vi "GUI_Scopes_NEW.vi"() -> ()   [LabVIEW 2020]
uses:
  Device Drivers/PXIdigitizer/subVis/Trigger.DigitalSource_TypDEf.ctl
  Device Drivers/ScopeAnalysis/SubVis/method_TypDef.ctl
  Device Drivers/ScopeAnalysis/SubVis/channels_TypDef.ctl
  Shared/GUI_Template/GUI_master/tcp new data cluster.ctl
  General-Controler/firstCall_TypDef.ctl
panel:
  in  "Trigger.Source::1":u16(ring) caption="Source"
  in  "Trigger.Coupling::1":u16(ring) caption="Coupling"
  in  "Analysis":T3={"Channel::1"=enum."Analysis1", "Calculations.Method::1"=enum."trigger", "Measurements::1"=-5e-07, "Calculations.Linked::1"=enum."na", "Calculations.Additional::1"=0.0} {"Calculations.Additional::1" min=0.0 max=0.0; "Measurements::1" min=0.0 max=0.0}
  in  "Horizontal.resolution::1":u16(ring) caption="Hres"
  in  "Horizontal.time_window::1":dbl=0.001 caption="TimeWindow" min=1e-09 max=100.0 format="%#_6p"
  in  "Horizontal.Min Sample Rate::1":dbl=500000000.0 caption="Sample Rate" min=1000.0 max=1000000000.0 step=1000000.0 format="%.0p"
  in  "Horizontal.Min Record Length::1":i32=1000 caption="Record Length" min=100 max=8388208 format="%.0p"
  in  "Trigger.Delay::1":dbl=0.5 caption="Delay" min=-10.0 max=10.0 format="%#_6p"
  in  "Trigger.Mode::1":u16(ring) caption="Mode"
  in  "Trigger.Low Level::1":dbl=0.5 caption="Level" min=-100.0 max=100.0 format="%#_6p"
  in  "Trigger.Slope::1":u16(ring) caption="Slope"
  in  "autoscale::1":bool caption="auto\nscale"
  in  "LocalSavingPath::1":path
  in  "save::1":bool=TRUE caption="save"
  in  "Select device":string(combo)="StagingPXIFast1"
  in  "Refresh Button":bool
  out "device status::1":string="Initialized" caption="Device status"
  in  "stop":bool=TRUE
  out "GUIdevice 1":string="StagingPXIFast1"
  in  "Waveform cluster":T4={"Channel::1"=enum."Channel0", "coupling::1"=1, "Impedance::1"=2, "offset::1"=0.0, "channelenabled::1"=1, "verticalrange::1"=0.1, "Names::1"="", "scopeTraceGUI::1"=[{"t0"=timestamp(-4.999999999588667e-07 s since 1904-01-01), "dt"=2e-09, "Y"=array[1000 elements]}, {"t0"=timestamp(-4.999999999588667e-07 s since 1904-01-01), "dt"=2e-09, "Y"=array[1000 elements]}]} {"verticalrange::1" min=0.0001 max=40.0 format="%_4f"; "channelenabled::1" items=["off", "on"]; "offset::1" min=-5.0 max=5.0}
  in  "Trigger.AnalogSource::1":T5(ring)=enum."External TRIG"
  in  "Trigger.DigitalSource::1":T6=enum."PFI 1"
  # "TRIGGER"
  # "HORIZONTAL"
  # "ANALYSIS"
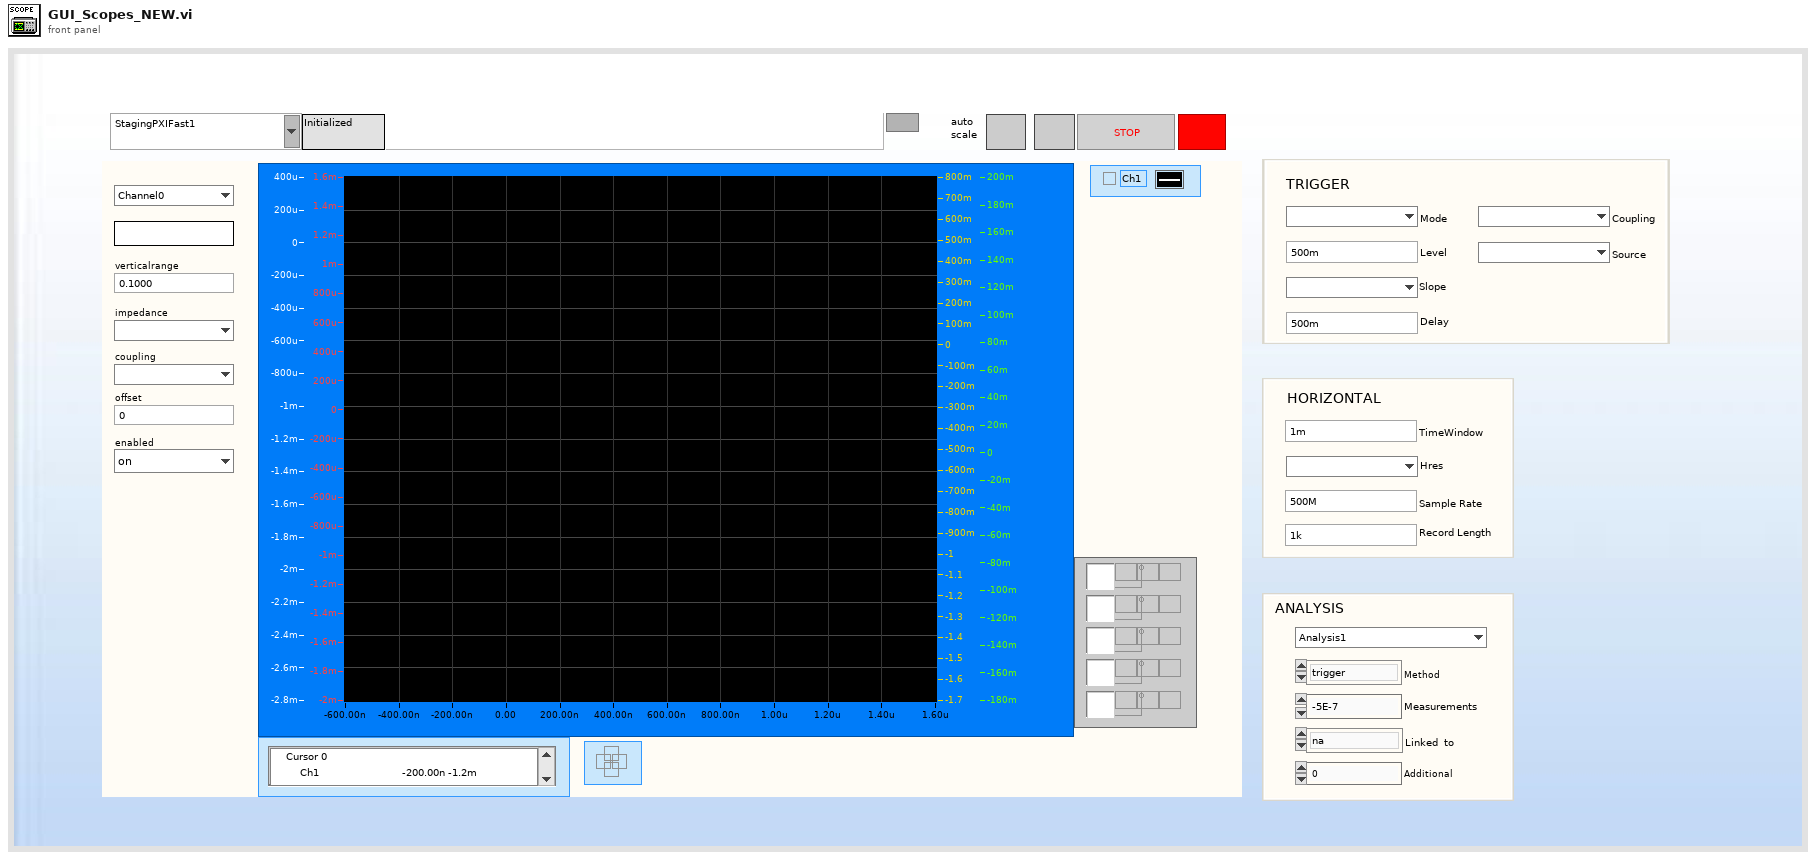
[diagram p1: front panel]
types:
  T1 = typedef "method_TypDef.ctl" = enum16{"n/a", "max", "min", "energy", "trigger", "maxtime", "mintime"}
  T2 = typedef "channels_TypDef.ctl" = enum16{"na", "StagingPXIFast1 scopeTrace.Channel0", "StagingPXIFast1 scopeTrace.Channel1", "StagingPXIFast2 scopeTrace.Channel0", "StagingPXIFast2 scopeTrace.Channel1", "StagingPXISlow scopeTrace.Channel0", "StagingPXISlow scopeTrace.Channel1", "StagingPXISlow scopeTrace.Channel2", "StagingPXISlow scopeTrace.Channel3", "StagingPXISlow scopeTrace.Channel4", "StagingPXISlow scopeTrace.Channel5", "StagingPXISlow scopeTrace.Channel6", "StagingPXISlow scopeTrace.Channel7"}
  T3 = cluster{"Channel::1":enum16{"Analysis1", "Analysis2", "Analysis3", "Analysis4", "Analysis5", "Analysis6", "Analysis7", "Analysis8", "Analysis9"}, "Calculations.Method::1":T1, "Measurements::1":dbl, "Calculations.Linked::1":T2, "Calculations.Additional::1":dbl}
  T4 = cluster{"Channel::1":enum16{"Channel0", "Channel1", "Channel2", "Channel3", "Channel4", "Channel5", "Channel6", "Channel7"}, "coupling::1":u16, "Impedance::1":u16, "offset::1":dbl, "channelenabled::1":u16, "verticalrange::1":dbl, "Names::1":string, "scopeTraceGUI::1":waveform(dbl)[]}
  T5 = enum16{"Channel 0", "Channel 1", "Channel 2", "Channel 3", "Channel 4", "Channel 5", "Channel 6", "Channel 7", "External TRIG"}
  T6 = typedef "Trigger.DigitalSource_TypDEf.ctl" = enum16{"RTSI 0", "RTSI 1", "RTSI 2", "RTSI 3", "RTSI 4", "RTSI 5", "RTSI 6", "PFI 0", "PFI 1", "PFI 2", "PXI Star Trigger"}
  T7 = typedef "tcp new data cluster.ctl" = cluster{"EventEnum":enum16{"new data", "connection status update"}, "Device name":string}
  T8 = typedef "firstCall_TypDef.ctl" = enum16{"reset", "read"}
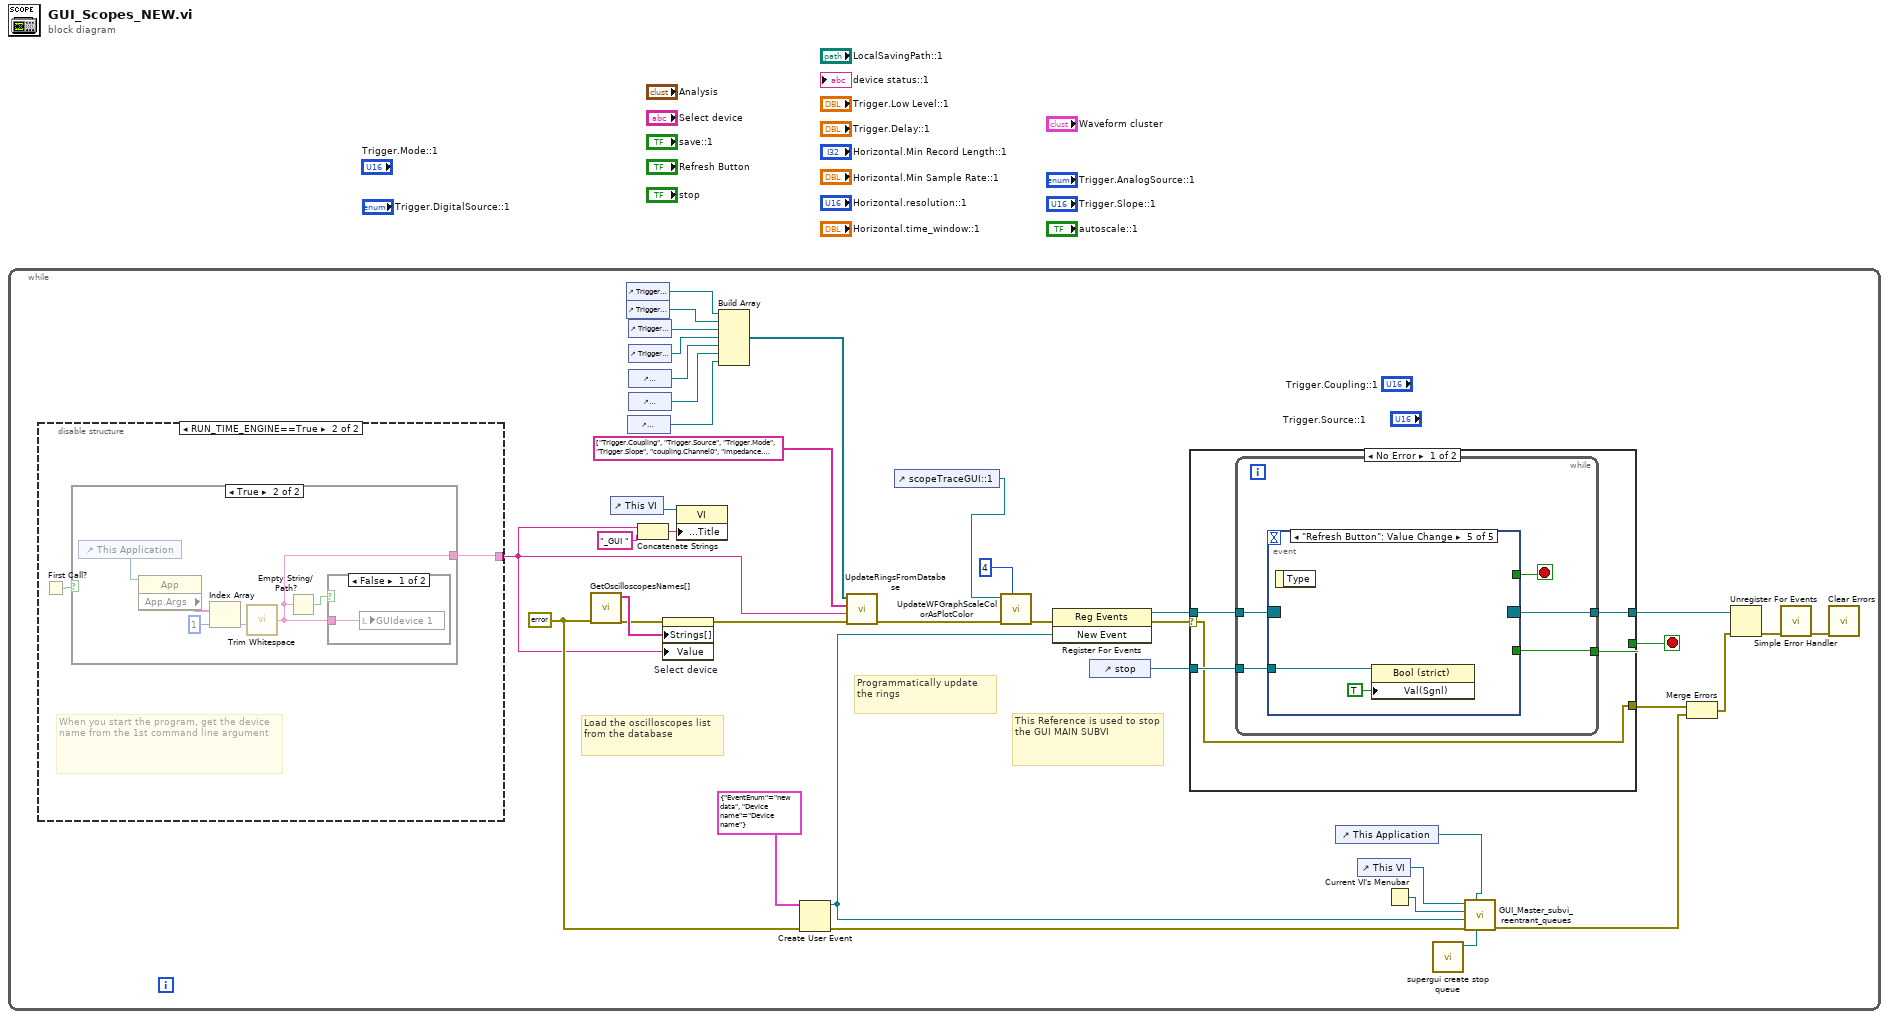
[diagram p0: block diagram]
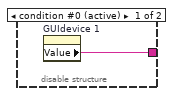
[diagram p2: hidden frame]
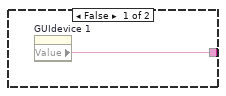
[diagram p3: hidden frame]
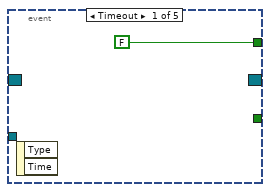
[diagram p5: hidden frame]
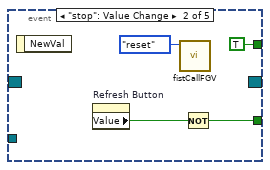
[diagram p6: hidden frame]
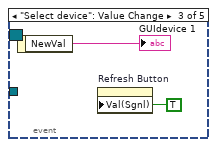
[diagram p7: hidden frame]
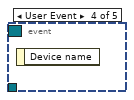
[diagram p8: hidden frame]
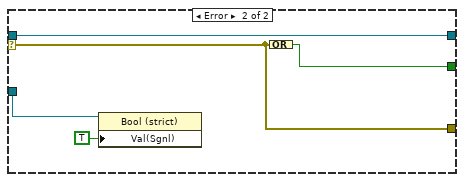
[diagram p9: hidden frame]
diagram:
  n1 = while {
    stop <- w36 stop-if-true
    w9 = errorcluster {"status"=FALSE, "code"=0, "source"=""} ("error in (no error)")
    # "Programmatically update the rings"
    # "Load the oscilloscopes list from the database"
    # "This Reference is used to stop the GUI MAIN SUBVI"
    n2 = disable-structure shown="RUN_TIME_ENGINE==True" {
      disable-tunnel: [w39 w40] -> w1
      frame condition #0 (active) {
        n3 = property on="GUIdevice 1" class="Str"() -> ("Value"=w39:string)  [unwired: 2 in, 2 out]
      }
      frame condition #1 {
        # "When you start the program, get the device name from the 1st command line argument"
        n4 = First Call?() -> (First Call?: T/F=w41:bool)
        n5 = case shown="True" w41 {
          tunnel: [w42 w43] -> w40
          frame False {
            n6 = property on="GUIdevice 1" class="Str"() -> ("Value"=w42:string)  [unwired: 2 in, 2 out]
          }
          frame True {
            n7 = control-ref of="This Application"() -> (w45:refnum<vi>)
            n8 = property class="App"(reference=w45) -> ("App.Args"=w46:string[])  [unwired: 1 in, 2 out]
            n9 = Index Array(array=w46, index=1) -> (element=w47:string)
            n10 = call <vilib>:"Trim Whitespace.vi"("string"=w47) -> ("trimmed string"=w43:string)  [unwired: 1 in]
            n11 = Empty String/Path?(string/path=w43) -> (empty?=w48:bool)
            n12 = case shown="False" w48 {
              tunnel: w43 -> [w49 _]
              frame False {
                n13 = local write "GUIdevice 1"(w49) -> ()
              }
              frame True {
              }
            }
          }
        }
      }
    }
    n14 = call "GetOscilloscopesNames[].vi"("error in (no error)"=w9) -> ("error IO"=w27:errorcluster, "OscilloscopesNames[]"=w28:string[])  [unwired: 9 in]
    n15 = control-ref of="This VI"() -> (w4:refnum<vi>)
    n16 = control-ref of="Trigger.Coupling::1"() -> (w7:refnum<vi>)
    n17 = control-ref of="Trigger.Source::1"() -> (w6:refnum<vi>)
    n18 = control-ref of="Horizontal.resolution::1"() -> (w8:refnum<vi>)
    n19 = control-ref of="Trigger.Mode::1"() -> (w25:refnum<vi>)
    n20 = control-ref of="Trigger.Slope::1"() -> (w24:refnum<vi>)
    n21 = control-ref of="coupling::1"() -> (w22:refnum<vi>)
    n22 = control-ref of="Impedance::1"() -> (w23:refnum<vi>)
    n23 = Concatenate Strings(w1, "_GUI ") -> (w3:string)
    n24 = property on="Select device" class="CmbBox"(error in=w27, "Strings[]"=w28, "Value"=w1) -> (error out=w26:errorcluster)  [unwired: 1 in, 1 out]
    n25 = property class="VI"(reference=w4, "Front Panel.Title"=w3) -> ()  [unwired: 1 in, 2 out]
    n26 = Build Array(w7, w6, w25, w24, w22, w23, w8) -> (w21:refnum<vi>[])
    n27 = Create User Event(user event datatype=T7 {"EventEnum"=enum."new data", "Device name"="Device name"} ("New Event"), error in=w9) -> (user event=w30:refnum<user-event>, error out=w31:errorcluster)
    n28 = call "UpdateRingsFromDatabase.vi"("error in (no error)"=w26, "device"=w1, "VariablesNames[]"=string[] ["Trigger.Coupling", "Trigger.Source", "Trigger.Mode", "Trigger.Slope", "coupling.Channel0", "impedance.Channel0", "Horizontal.resolution"], "RingsRefs[]"=w21) -> ("error out"=w18:errorcluster)  [unwired: 7 in]
    n29 = control-ref of="scopeTraceGUI::1"() -> (w12:refnum<vi>)
    n30 = call "UpdateWFGraphScaleColorAsPlotColor.vi"("Plots#"=4, "error in (no error)"=w18, "WaveformGraph in"=w12) -> ("error out"=w17:errorcluster)  [unwired: 8 in]
    n31 = register-events(error in=w17, w30) -> (reference out=w38:refnum<event-registration>, error out=w16:errorcluster)  [unwired: 1 in]
    n32 = control-ref of="stop"() -> (w35:refnum<vi>)
    n33 = case shown="No Error" w16 {
      selector: w16 -> [w50 w69]
      tunnel: w38 -> [w54 w71]
      tunnel: [w53 w71] -> w37
      tunnel: [w52 w70] -> w36
      tunnel: w35 -> [w51 w72]
      tunnel: [w50 w69] -> w14
      frame No Error {
        n34 = while {
          tunnel: w54 -> [w59]
          tunnel: [w58] -> w53
          tunnel: [w56] -> w52
          tunnel: w51 -> [w55]
          stop <- w57 stop-if-true
          n35 = event shown="[4] \"Refresh Button\": Value Change" {
            selector: w59 -> [_ _ _ _ _]
            dyn-events: [_ _ _ _ _] -> w58
            timeout: _ -> [_ _ _ _ _]
            tunnel: [FALSE TRUE _ _ _] -> w57
            tunnel: [_ w62 _ _ _] -> w56
            tunnel: w55 -> [_ _ _ _ w68]
            event Timeout {
              n36 = event-data() -> ()  [unwired: 1 in, 2 out]
            }
            event "stop": Value Change {
              n37 = event-data() -> ()  [unwired: 1 in, 1 out]
              n38 = property on="Refresh Button" class="Bool (strict)"() -> ("Value"=w63:bool)  [unwired: 2 in, 2 out]
              n39 = call "fistCallFGV.vi"("Function"=firstCall_TypDef."reset") -> ()  [unwired: 9 in, 2 out]
              n40 = Not(x=w63) -> (.not. x?=w62:bool)
            }
            event "Select device": Value Change {
              n41 = event-data() -> ("NewVal"=→"GUIdevice 1":string)  [unwired: 1 in]
              n42 = property on="Refresh Button" class="Bool (strict)"("Val(Sgnl)"=TRUE ("Value (Signaling)")) -> ()  [unwired: 2 in, 2 out]
            }
            event User Event {
              n43 = event-data() -> ()  [unwired: 1 in, 1 out]
            }
            event "Refresh Button": Value Change {
              n44 = event-data() -> ()  [unwired: 1 in, 1 out]
              n45 = property class="Bool (strict)"(reference=w68, "Val(Sgnl)"=TRUE ("Value (Signaling)")) -> ()  [unwired: 1 in, 2 out]
            }
          }
        }
      }
      frame Error {
        n46 = property class="Bool (strict)"(reference=w72, "Val(Sgnl)"=TRUE ("Value (Signaling)")) -> ()  [unwired: 1 in, 2 out]
        n47 = Compound Arithmetic op=OR(w69) -> (w70:bool)
      }
    }
    n48 = control-ref of="This Application"() -> (w29:refnum<vi>)
    n49 = control-ref of="This VI"() -> (w34:refnum<vi>)
    n50 = Current VI's Menubar() -> (w33:refnum<k9>)
    n51 = call "supergui create stop queue.vi"() -> ("STOP Queue out"=w5:refnum<queue>)  [unwired: 11 in]
    n52 = call "GUI_Master_subvi_reentrant_queues.vi"("STOP Queue in"=w5, "This Application"=w29, "error in (no error)"=w31, "tcp data event"=w30, "Caller menu reference"=w33, "Caller VI ref"=w34) -> ("error out"=w15:errorcluster)  [unwired: 5 in]
    n53 = Merge Errors(w14, w15) -> (w13:errorcluster)
    n54 = Unregister For Events(event registration refnum=w37, error in=w13) -> (error out=w11:errorcluster)
    n55 = call <vilib>:"Simple Error Handler.vi"("error in (no error)"=w11) -> ("error out"=w10:errorcluster)  [unwired: 4 in, 4 out]
    n56 = call <vilib>:"Clear Errors.vi"("error in (no error)"=w10) -> ()  [unwired: 5 in, 2 out]
  }
